vi "Open Driver-Defined Property.vi"(0 "session in":refnum<k21>, 7 "property in":refnum<k21>, 11 "error in (no error)":errorcluster) -> (4 "session out":refnum<k21>, 8 "property out":refnum<k21>, 15 "error out":errorcluster)   [LabVIEW 2020, in "SLSC.lvlib"]
doc: "Opens a reference to a driver-defined property. This allows the application to programmatically get information about the property at run time. The SLSC Property I/O control does not display driver-defined properties, but you can type them into the I/O control or use System » API Reflection properties such as Sys.DeviceProperties to query their names."
uses:
  <vilib>/SLSC/SLSC.lvlib
  nislsclvapi.dll
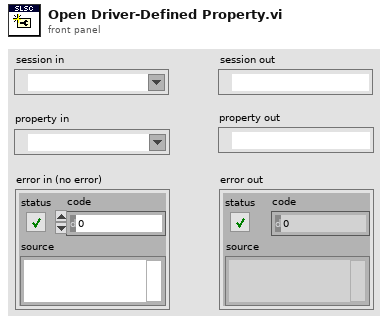
[diagram p1: front panel]
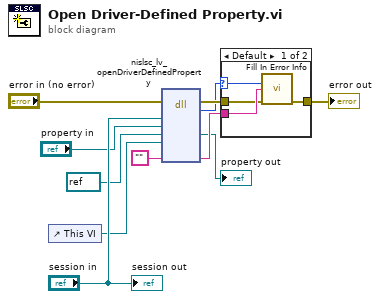
[diagram p0: block diagram]
diagram:
  n1 = control-ref of="This VI"() -> (w1:refnum<vi>)
  n2 = dll-call lib="nislsclvapi.*" fn="nislsc_lv_openDriverDefinedProperty"(error in="error in (no error)", "session"="session in", "propertyIn"="property in", "propertyRefObjOut"=refnum<k21> refnum ("property out"), "lvAppRef"=w1, "extendedErrorInfo"="") -> (error out=w8:errorcluster, "return type"=w7:i32, "propertyRefObjOut"=→"property out":refnum<k21>, "extendedErrorInfo"=w9:string)  [unwired: 7 in, 1 out]
  n3 = case shown="Default" w7 {
    selector: w7 -> [w15 _]
    tunnel: w9 -> [w14 _]
    tunnel: w8 -> [w13 w16]
    tunnel: [w12 w16] -> w6
    frame Default {
      n4 = call <vilib>:"Fill In Error Info.vi"("status code"=w15, "extended error info"=w14, "error in"=w13) -> ("error out"=w12:errorcluster)  [unwired: 12 in]
    }
    frame 0 {
    }
  }
  "error out" <- w6
  "session out" <- "session in"
